vi "Periodic Tasks.vi"(8 "Error In":errorcluster) -> ()   [LabVIEW 2012]
doc: "This VI runs in parallel to other tasks. It can contain as many user-defined periodic loops as you need. These can carry out PID or other sorts of timed response."
uses:
  Controls/Sensor.ctl
  Globals/Jaguar Commands.vi
  Globals/Robot Jaguars.vi
  Globals/Potentiometers.vi
  Globals/Max Steer Voltage.vi
  Globals/DriveSystemMode.vi
  <vilib>/Rock Robotics/WPI/Joystick/WPI_JoystickGetSetRefNum.vi
  Globals/Calculated Shooter Speed.vi
  Globals/Image Height.vi
  Globals/Alignment Error.vi
panel:
  in  "Axis 3":dbl
  out "axis 3 (throttle)":dbl
  out "Multiplier":dbl
  in  "Post speed gain":dbl=0.23
  out "Motor Output":dbl=-0.0479915163000006
  out "Center of Mass X 2":dbl(graph)
  in  "reinitialize? (F)":bool=TRUE
  out "Laser Broken?":bool=TRUE
  out "Actuator Position":dbl=2.584470945
  out "Raw String from UDP":string="!195,#END"
  out "Aiming Error":dbl=-320.0
  in  "Center of Mass X":dbl
  in  "Invert":bool=TRUE
  in  "PID gains":T1={"proportional gain (Kc)"=0.0076, "integral time (Ti, min)"=0.0, "derivative time (Td, min)"=0.0031} {"derivative time (Td, min)" format="%.6f"; "integral time (Ti, min)" format="%.9f"; "proportional gain (Kc)" format="%.6f"}
  in  "PID gains (actuator)":T1={"proportional gain (Kc)"=1.95, "integral time (Ti, min)"=0.0, "derivative time (Td, min)"=0.0} {"derivative time (Td, min)" format="%.6f"; "integral time (Ti, min)" format="%.3f"; "proportional gain (Kc)" format="%.3f"}
  in  "PID gains (weak motor)":T1={"proportional gain (Kc)"=8.0, "integral time (Ti, min)"=0.0, "derivative time (Td, min)"=0.0} {"derivative time (Td, min)" format="%.6f"; "integral time (Ti, min)" format="%.3f"; "proportional gain (Kc)" format="%.3f"}
  in  "PID gains (strong motor)":T1={"proportional gain (Kc)"=4.0, "integral time (Ti, min)"=0.0, "derivative time (Td, min)"=0.0} {"derivative time (Td, min)" format="%.6f"; "integral time (Ti, min)" format="%.3f"; "proportional gain (Kc)" format="%.3f"}
  # "Steers"
  # "Steering"
  # "Actuator"
  # "Shooter"
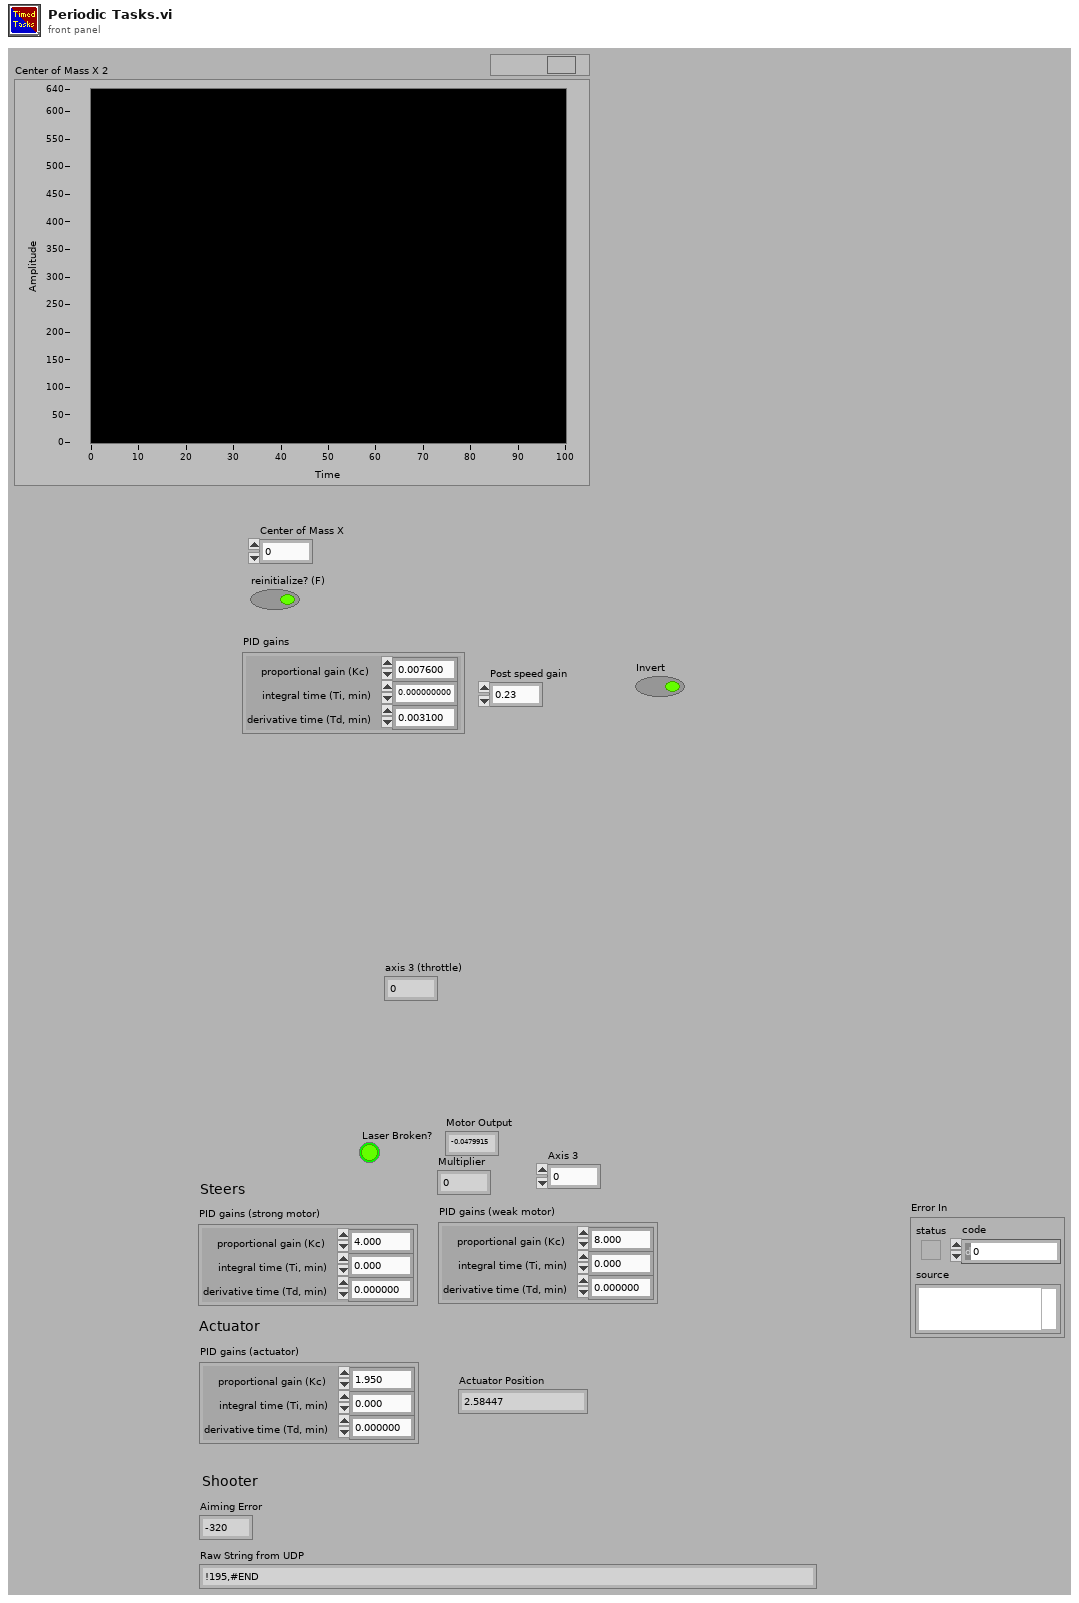
[diagram p1: front panel]
types:
  T1 = cluster{"proportional gain (Kc)":dbl, "integral time (Ti, min)":dbl, "derivative time (Td, min)":dbl}
  T2 = typedef "WPI_JoystickDevRef.ctl" = cluster{"Device":T3}
  T3 = typedef "WPI_JoystickDeviceEnum.ctl" = enum16{"USB 1", "USB 2", "USB 3", "USB 4", "Kinect 1", "Kinect 2"}
  T4 = typedef "WPI_JoystickButtonState.ctl" = cluster{"Button 1":bool, "Button 2":bool, "Button 3":bool, "Button 4":bool, "Button 5":bool, "Button 6":bool, "Button 7":bool, "Button 8":bool, "Button 9":bool, "Button 10":bool, "Button 11":bool, "Button 12":bool}
  T5 = typedef "Sensor.ctl" = enum16{"Potentiometer", "Encoder"}
  T6 = typedef "Drive System Mode.ctl" = enum16{"Normal", "Crab", "Shoot"}
  T7 = typedef "WPI_AnalogChannelDevRef.ctl" = cluster{"DevStatus":errorcluster, "Analog Module":T8, "Analog Channel":T9}
  T8 = typedef "FPGA_TypedefAnalogModule.ctl" = enum16{"Analog Module 1", "Analog Module 2"}
  T9 = typedef "FPGA_AIChannel.ctl" = enum8{"AI 1", "AI 2", "AI 3", "AI 4", "AI 5", "AI 6", "AI 7", "AI 8", "Invalid"}
  T10 = cluster{"Front Left":T7, "Front Right":T7, "Rear Left":T7, "Rear Right":T7, "Actuator":T7}
  T11 = typedef "WPI_MotorControlDeviceRef.ctl" = cluster{"DeviceStatus":errorcluster, "Type":enum16{"PWM", "CAN"}, "PWM":cluster{"Digital Module":T12, "PWM Channel":T13, "DeadBand":T14}, "CAN":cluster{"Device Number":u8, "Control Mode":T15, "Semaphore":T16, "Max Vout":dbl}, "Invert":bool, "TransformRef":T17, "InvTransformRef":T17}
  T12 = typedef "FPGA_TypedefDigitalModule.ctl" = enum16{"Digital Module 1", "Digital Module 2"}
  T13 = typedef "FPGA_DIOPWMChannel.ctl" = enum8{"PWM 1", "PWM 2", "PWM 3", "PWM 4", "PWM 5", "PWM 6", "PWM 7", "PWM 8", "PWM 9", "PWM 10", "Invalid"}
  T14 = typedef "WPI_PWMDeadband.ctl" = cluster{"Name":string, "maxPositivePwm":i32, "minPositivePwm":i32, "centerPwm":i32, "maxNegativePwm":i32, "minNegativePwm":i32, "angularRange":u16}
  T15 = typedef "WPI_CANJaguar_ControlMode.ctl" = enum8{"Percent VBus", "Current", "Speed", "Position", "Voltage"}
  T16 = typedef "Semaphore RefNum" = refnum<k1>
  T17 = typedef "WPI_PWMTransform_ConPane.ctl" = refnum<vi>
  T18 = cluster{"Front Left Drive":T11, "Front Right Drive":T11, "Rear Left Drive":T11, "Rear Right Drive":T11, "Front Left Steer":T11, "Front Right Steer":T11, "Rear Left Steer":T11, "Rear Right Steer":T11}
  T19 = cluster{"axis 1 (x)":dbl, "axis 2 (y)":dbl, "axis 3 (throttle)":dbl, "axis 4":dbl, "axis 5":dbl, "axis 6":dbl}
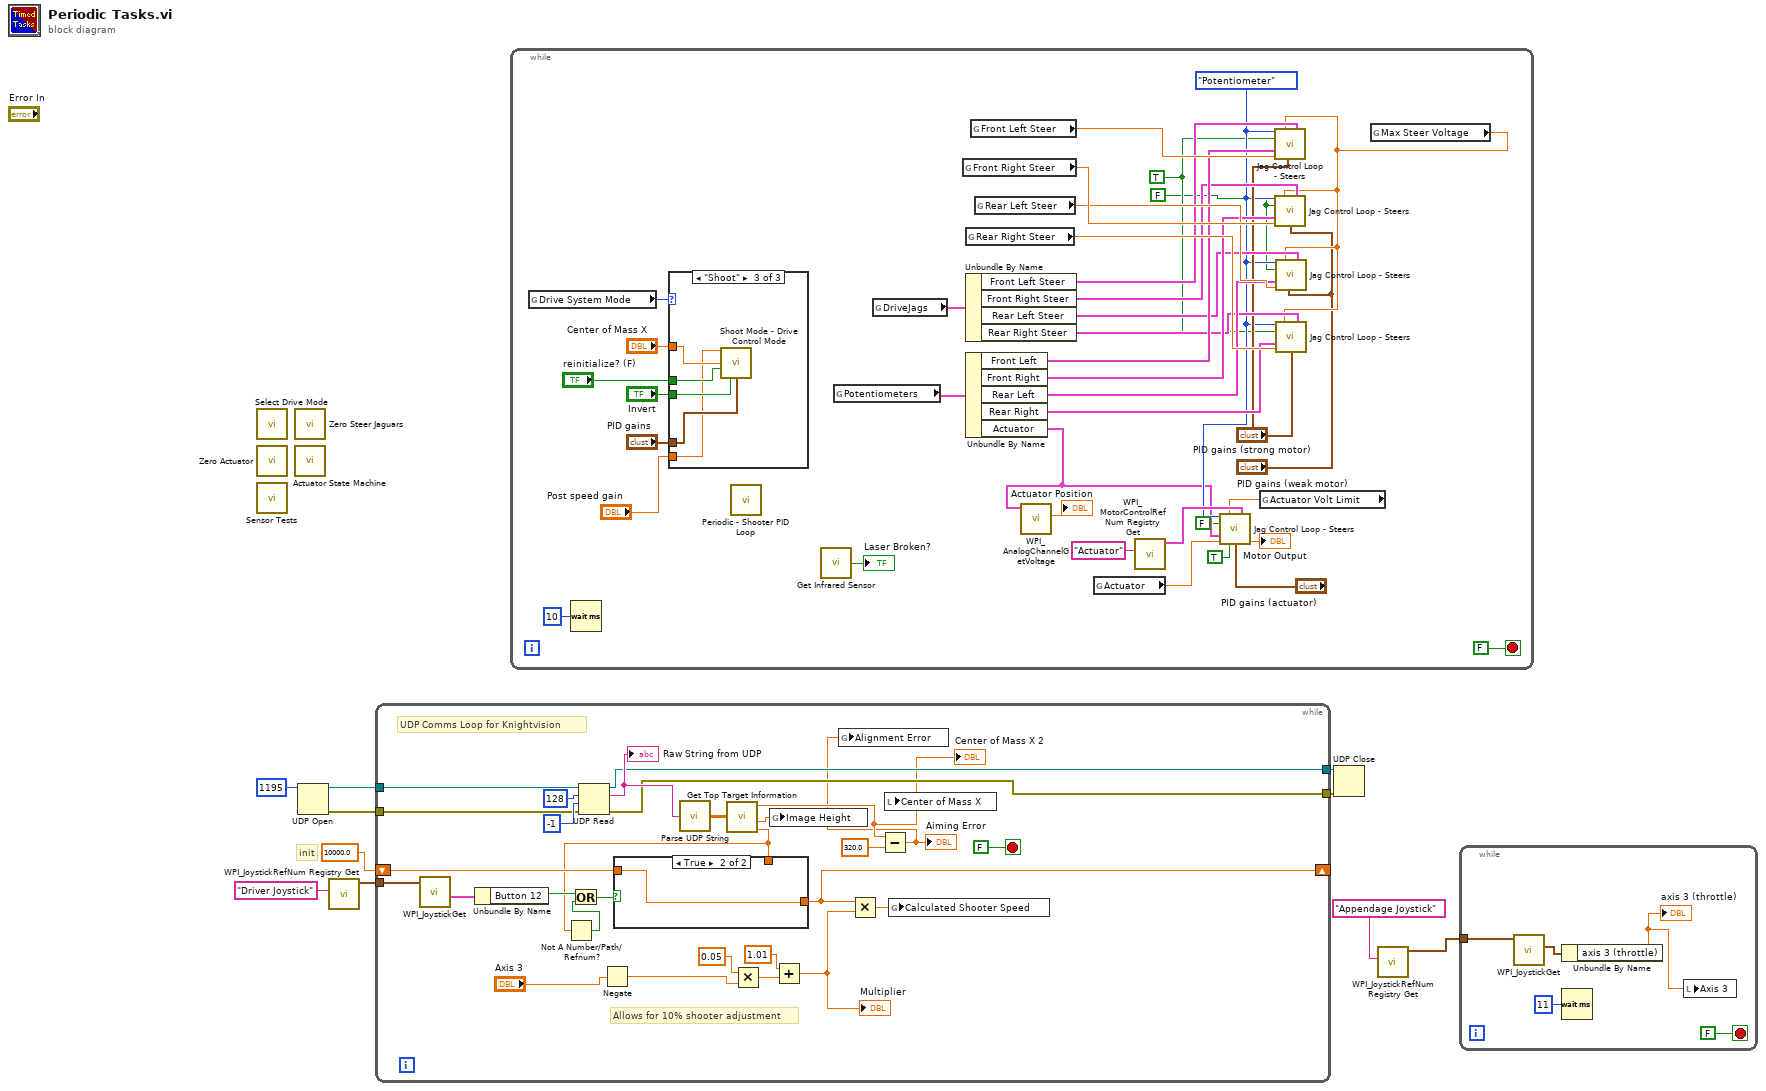
[diagram p0: block diagram]
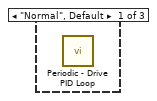
[diagram p3: hidden frame]
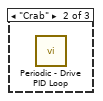
[diagram p4: hidden frame]
diagram:
  # "init"
  n1 = call "Select Drive Mode.vi"() -> ()  [unwired: 12 in]
  n2 = call "Zero Actuator.vi"() -> ()  [unwired: 12 in]
  n3 = call "Sensor Tests.vi"() -> ()  [unwired: 12 in]
  n4 = call "Zero Steer Jaguars.vi"() -> ()  [unwired: 12 in]
  n5 = call "Actuator State Machine.vi"() -> ()  [unwired: 1 in]
  n6 = UDP Open(11:u16 1195 ("port")) -> (port=w9:refnum<k16>, 0:w8:errorcluster)  [unwired: 4 in, 1 out]
  n7 = call <vilib>:"WPI_JoystickRefNum Registry Get.vi"("refnum name"="Driver Joystick") -> ("JoystickDevRef"=w4:T2)  [unwired: 9 in, 1 out]
  n8 = while {
    tunnel: w9 -> [w32]
    tunnel: w8 -> [w31]
    tunnel: [w30] -> w7
    tunnel: [w29] -> w6
    shift-right: [w17] -> _
    shift-left: 10000.0 ("Calculated Shooter Speed") -> [w27]
    tunnel: w4 -> [w25]
    stop <- FALSE stop-if-true
    # "Allows for 10% shooter adjustment"
    # "UDP Comms Loop for Knightvision"
    n9 = call <vilib>:"WPI_JoystickGet.vi"("JoystickDevRef"=w25) -> ("Buttons"=w26:T4)  [unwired: 4 in, 2 out]
    n10 = Unbundle By Name(w26) -> ("Button 12"=w22:bool)
    n11 = UDP Read(connection ID=w32, max size (548)=128, timeout ms (25000)=-1, 8:w31) -> (data out=w37:string, error out=w29:errorcluster, 3:w30:refnum<k16>)  [unwired: 2 out]
    "Raw String from UDP" <- w37
    n12 = Negate(x="Axis 3") -> (-x=w12:dbl)
    n13 = call "Parse UDP String.vi"("UDP Packet In"=w37) -> ("Array"=w34:dbl[][])
    n14 = call "Get Top Target Information.vi"("Vision Info Array"=w34) -> ("Center of Mass X"=w28:dbl, "Bounding Box Height"=w23:dbl, "Calculated Shooter Speed"=w20:dbl)  [unwired: 1 out]
    "Center of Mass X 2" <- w28
    n15 = Not A Number/Path/Refnum?(number/path/refnum=w20) -> (NaN/Path/Refnum?=w19:bool)
    n16 = Or(x=w22, y=w19) -> (x .or. y?=w21:bool)
    n17 = case shown="True" w21 {
      tunnel: w20 -> [w39 _]
      tunnel: [w39 w40] -> w17
      tunnel: w27 -> [_ w40]
      frame False {
      }
      frame True {
      }
    }
    n18 = Multiply(x=0.05, y=w12) -> (x*y=w14:dbl)
    n19 = global write "Image Height.vi" "Image Height"(w23) -> ()
    n20 = Add(x=1.01, y=w14) -> (x+y=w15:dbl)
    "Multiplier" <- w15
    n21 = Multiply(x=w17, y=w15) -> (x*y=w18:dbl)
    n22 = Subtract(x=w28, y=320.0) -> (x-y=w24:dbl)
    "Aiming Error" <- w24
    n23 = global write "Alignment Error.vi" "Alignment Error"(w24) -> ()
    n24 = local write "Center of Mass X"(w28) -> ()
    n25 = global write "Calculated Shooter Speed.vi" "Calculated Shooter Speed"(w18) -> ()
  }
  n26 = while {
    stop <- FALSE stop-if-true
    w43 = FALSE ("Strong wheel?")
    w44 = TRUE
    w57 = Sensor."Potentiometer" ("Sensor")
    n27 = global read "DriveSystemMode.vi" "Drive System Mode"() -> (w51:T6)
    n28 = Wait (ms)(milliseconds to wait=u32 10) -> ()  [unwired: 1 out]
    n29 = case shown="\"Shoot\"" w51 {
      tunnel: "PID gains" -> [_ _ w84]
      tunnel: "Invert" -> [_ _ w83]
      tunnel: "Center of Mass X" -> [_ _ w82]
      tunnel: "reinitialize? (F)" -> [_ _ w81]
      tunnel: "Post speed gain" -> [_ _ w80]
      frame "Normal", Default {
        n30 = call "Periodic - Drive PID Loop.vi"() -> ()  [unwired: 12 in]
      }
      frame "Crab" {
        n31 = call "Periodic - Drive PID Loop.vi"() -> ()  [unwired: 12 in]
      }
      frame "Shoot" {
        n32 = call "Shoot Mode - Drive Control Mode.vi"("Post Speed Limit"=w80, "Center of Mass X"=w82, "reinitialize? (F)"=w81, "Invert"=w83, "PID gains"=w84) -> ()  [unwired: 11 in]
      }
    }
    n33 = call "Periodic - Shooter PID Loop.vi"() -> ()  [unwired: 1 in]
    n34 = call "Get Infrared Sensor.vi"() -> ("Laser Broken?"=→"Laser Broken?":bool)
    n35 = global read "Potentiometers.vi" "Potentiometers"() -> (w72:T10)
    n36 = global read "Robot Jaguars.vi" "DriveJags"() -> (w77:T18)
    n37 = global read "Jaguar Commands.vi" "Front Right Steer"() -> (w75:dbl)
    n38 = global read "Jaguar Commands.vi" "Rear Right Steer"() -> (w73:dbl)
    n39 = Unbundle By Name(w77) -> ("Front Left Steer"=w67:T11, "Front Right Steer"=w66:T11, "Rear Left Steer"=w65:T11, "Rear Right Steer"=w64:T11)
    n40 = Unbundle By Name(w72) -> ("Front Left"=w71:T7, "Front Right"=w70:T7, "Rear Left"=w69:T7, "Rear Right"=w68:T7, "Actuator"=w53:T7)
    n41 = global read "Jaguar Commands.vi" "Front Left Steer"() -> (w76:dbl)
    n42 = global read "Jaguar Commands.vi" "Rear Left Steer"() -> (w74:dbl)
    n43 = call <vilib>:"WPI_AnalogChannelGetVoltage.vi"("AIDeviceRef"=w53) -> ("Voltage"=→"Actuator Position":dbl)  [unwired: 8 in, 2 out]
    n44 = global read "Jaguar Commands.vi" "Actuator"() -> (w55:dbl)
    n45 = call <vilib>:"WPI_MotorControlRefNum Registry Get.vi"("refnum name"="Actuator") -> ("MotorControlDevRef"=w58:T11)  [unwired: 9 in, 1 out]
    n46 = global read "Jaguar Commands.vi" "Actuator Volt Limit"() -> (w54:dbl)
    n47 = call "Jag Control Loop - Steers.vi"("Sensor"=w57, "Voltage Limit"=w54, "MotorControlDevRef"=w58, "Strong wheel?"=FALSE, "AIDeviceRef"=w53, "Command"=w55, "Invert"=TRUE, "PID gains"="PID gains (actuator)") -> ("Motor Output"=→"Motor Output":dbl)  [unwired: 6 in, 1 out]
    n48 = global read "Max Steer Voltage.vi" "Max Steer Voltage"() -> (w63:dbl)
    n49 = call "Jag Control Loop - Steers.vi"("Sensor"=w57, "Voltage Limit"=w63, "MotorControlDevRef"=w67, "Strong wheel?"=w44, "AIDeviceRef"=w71, "Command"=w76, "PID gains"="PID gains (strong motor)") -> ()  [unwired: 7 in, 2 out]
    n50 = call "Jag Control Loop - Steers.vi"("Sensor"=w57, "Voltage Limit"=w63, "MotorControlDevRef"=w66, "Strong wheel?"=w43, "AIDeviceRef"=w70, "Command"=w75, "PID gains"="PID gains (weak motor)") -> ()  [unwired: 7 in, 2 out]
    n51 = call "Jag Control Loop - Steers.vi"("Sensor"=w57, "Voltage Limit"=w63, "MotorControlDevRef"=w65, "Strong wheel?"=w43, "AIDeviceRef"=w69, "Command"=w74, "PID gains"="PID gains (weak motor)") -> ()  [unwired: 7 in, 2 out]
    n52 = call "Jag Control Loop - Steers.vi"("Sensor"=w57, "Voltage Limit"=w63, "MotorControlDevRef"=w64, "Strong wheel?"=w44, "AIDeviceRef"=w68, "Command"=w73, "PID gains"="PID gains (strong motor)") -> ()  [unwired: 7 in, 2 out]
  }
  n53 = UDP Close(connection ID=w7, 8:w6) -> ()  [unwired: 2 out]
  n54 = call <vilib>:"WPI_JoystickRefNum Registry Get.vi"("refnum name"="Appendage Joystick") -> ("JoystickDevRef"=w1:T2)  [unwired: 9 in, 1 out]
  n55 = while {
    tunnel: w1 -> [w88]
    stop <- FALSE stop-if-true
    n56 = call <vilib>:"WPI_JoystickGet.vi"("JoystickDevRef"=w88) -> ("Axes"=w89:T19)  [unwired: 4 in, 2 out]
    n57 = Unbundle By Name(w89) -> ("axis 3 (throttle)"=w85:dbl)
    "axis 3 (throttle)" <- w85
    n58 = Wait (ms)(milliseconds to wait=u32 11) -> ()  [unwired: 1 out]
    n59 = local write "Axis 3"(w85) -> ()
  }
